vi "Get Drive Type.vi"(3 "error in (no error)":errorcluster, 5 "Root Path name (C:\\)":string="c:\\") -> (0 "error out":errorcluster, 1 "Dup Root Path name (C:\\)":string="c:\\", 2 "Drive Type":T1(ring))   [LabVIEW 2011, in "API.lvlib"]
doc: "Retrieves the type of the requested drive.\nMay be one of the following....\n0:Unkown\n1:No Root\n2:Removable\n3:Fixed\n4:Remote\n5:CD Rom\n6:Ramdisk"
uses:
  API.lvlib
  kernel32.dll
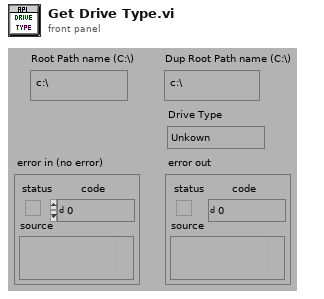
[diagram p1: front panel]
types:
  T1 = enum16{"Unkown", "No Root", "Removable", "Fixed", "Remote", "CD Rom", "Ramdisk"}
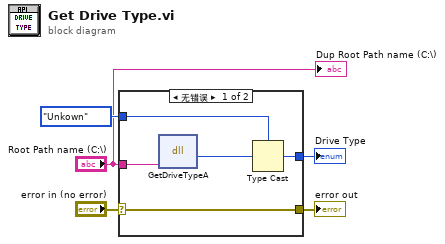
[diagram p0: block diagram]
diagram:
  n1 = case shown="无错误" "error in (no error)" {
    selector: "error in (no error)" -> [w6 w11]
    tunnel: "Root Path name (C:\\)" -> [w10 _]
    tunnel: [w7 w12] -> w4
    tunnel: T1."Unkown" ("Drive Type") -> [w8 w12]
    tunnel: [w6 w11] -> w1
    frame No Error {
      n2 = dll-call lib="kernel32.dll" fn="GetDriveTypeA" label="GetDrive Type"("lpRootPathName"=w10) -> (w9:u16)  [unwired: 4 in, 2 out]
      n3 = Type Cast(type=w8, x=w9) -> (*(type *) &x=w7:T1)
    }
    frame Error {
    }
  }
  "Drive Type" <- w4
  "error out" <- w1
  "Dup Root Path name (C:\\)" <- "Root Path name (C:\\)"
